vi "Update Monkeys Status.vi"(6 "Overwrite":bool, 7 "In ALL?":bool, 8 "error in (no error)":errorcluster, 9 "Status":T1, 10 "Monkey ID":string, 11 "Tamer in":refnum<class "Tamer.lvclass">=refnum) -> (0 "error out":errorcluster, 3 "Tamer out":refnum<class "Tamer.lvclass">)   [LabVIEW 2020, in "CIRCUS_uServices.lvlib" / "Tamer.lvlib" / "Tamer.lvclass"]
uses:
  Tamer.lvclass
  Monkey Summary.ctl
  Link Chain GUI.ctl
  TALOS/TALOS_PPL.lvlibp/Father of all uServices/Father of all uServices/Father of all uServices.lvclass
  TALOS/TALOS_PPL.lvlibp
  Run Utilities/TypeDefs/Monkey Status.ctl
  Run Utilities/Run Utilities.lvlib
  TALOS/TALOS_PPL.lvlibp/Father of all uServices/Father of all uServices/Children Methods/Get GUI Item Value - Variant.vi
  C:/Users/marco/Documents/GitHub_Lab/CIRCUS/TALOS/TALOS_PPL.lvlibp/Father of all uServices/Father of all uServices/Father of all uServices.lvclass
  C:/Users/marco/Documents/GitHub_Lab/CIRCUS/TALOS/TALOS_PPL.lvlibp/Ancestor/Ancestor/Ancestor.lvclass
  C:/Users/marco/Documents/GitHub_Lab/CIRCUS/TALOS/Actor Framework.lvlibp/1abvi3w/vi.lib/ActorFramework/Actor/Actor.lvclass
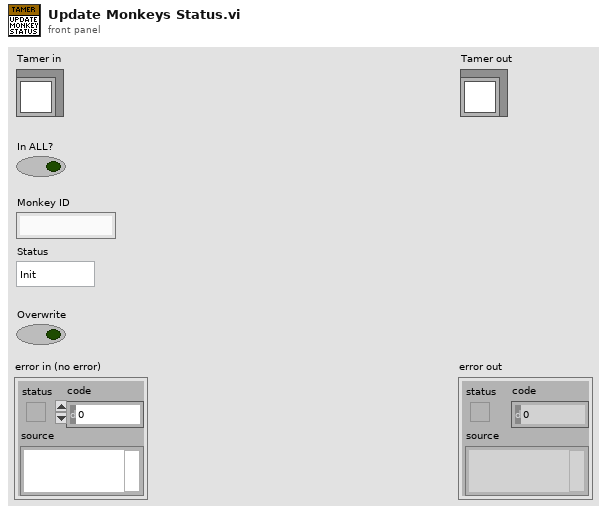
[diagram p1: front panel]
types:
  T1 = typedef "CIRCUS_uServices.lvlib/Run Utilities.lvlib/Monkey Status.ctl" = enum16{"Init", "Paused", "Ongoing", "Stopped", "Finished (no errors)", "Finished (with errors)"}
  T2 = typedef "CIRCUS_uServices.lvlib/Tamer.lvlib/Tamer.lvclass/Monkey Summary.ctl" = cluster{"Color":u32, "Status":T1, "Continuous":bool, "Scripts left":u32, "Scripts skipped":u32, "ETA":string, "Current Action":string, "Report from previous RUNs":string, "Monkey ID":string, "With DAQ?":bool, "Linked?":T3, "Paused":bool}
  T3 = typedef "CIRCUS_uServices.lvlib/Tamer.lvlib/Tamer.lvclass/Link Chain GUI.ctl" = bool
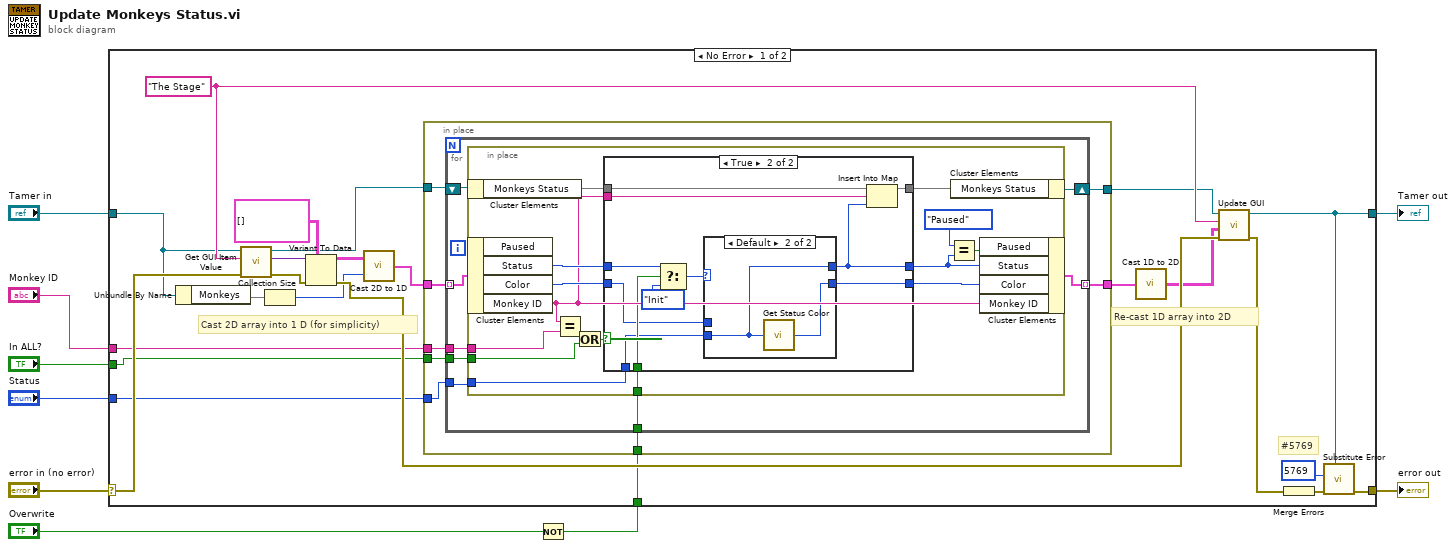
[diagram p0: block diagram]
diagram:
  n1 = Not(x="Overwrite") -> (.not. x?=w1:bool)
  n2 = case shown="No Error" "error in (no error)" {
    selector: "error in (no error)" -> [w28 w84]
    tunnel: [w33 w84] -> w8
    tunnel: [w32 w83] -> w6
    tunnel: "Tamer in" -> [w10 w83]
    tunnel: "Status" -> [w16 _]
    tunnel: "Monkey ID" -> [w15 _]
    tunnel: "In ALL?" -> [w14 _]
    tunnel: w1 -> [w11 _]
    frame No Error {
      w17 = "The Stage" ("FP Item Name")
      # "Re-cast 1D array into 2D"
      # "Cast 2D array into 1 D (for simplicity)"
      # "#5769"
      n3 = Unbundle By Name(w10) -> ("Monkeys"=w21:map{string, string[]})
      n4 = call-poly "Get GUI Item Value.vi"("error in (no error)"=w28, "FP Item Name"=w17, "uService Template in"=w10) -> ("error out"=w22:errorcluster, "Value"=w24:variant, "uService Template out"=w13:refnum<class "Tamer.lvclass">)  [unwired: 6 in]
      n5 = Collection Size(1:w21) -> (0:w20:i32)
      n6 = Variant To Data(error in=w22, type=T2[][] [] ("2D Synchronous Monkeys"), Variant=w24) -> (data=w23:T2[][], error out=w26:errorcluster)
      n7 = call "Cast 2D to 1D.vi"("1D size"=w20, "2D Synchronous Monkeys"=w23) -> ("1D Synchronous Monkeys"=w27:T2[])
      n8 = in-place {
        in-place-border: w27 -> [w41]
        in-place-border: [w40] -> w25
        in-place-border: w16 -> [w37]
        in-place-border: w15 -> [w39]
        in-place-border: w14 -> [w38]
        in-place-border: w13 -> [w36]
        in-place-border: [w35] -> w12
        in-place-border: w11 -> [w34]
        n9 = for {
          tunnel: w41 -> [w49] mode=indexing
          tunnel: w37 -> [w48]
          tunnel: [w47] -> w40 mode=indexing
          tunnel: w39 -> [w46]
          tunnel: w38 -> [w45]
          shift-right: [w43] -> w35
          shift-left: w36 -> [w44]
          tunnel: w34 -> [w42]
          n10 = in-place {
            in-place-border: w48 -> [w64]
            in-place-border: w46 -> [w63]
            in-place-border: w45 -> [w60]
            in-place-border: w42 -> [w53]
            n11 = in-place-cluster #1(w44) -> ("Monkeys Status"=w56:map{string, T1})
            n12 = in-place-cluster #2(w49) -> ("Status"=w59:T1, "Color"=w57:u32, "Monkey ID"=w54:string)  [unwired: 1 out]
            n13 = Equal?(x=w54, y=w63) -> (x = y?=w61:bool)
            n14 = Or(x=w61, y=w60) -> (x .or. y?=w62:bool)
            n15 = case shown="True" w62 {
              tunnel: [w66 w70] -> w58
              tunnel: w64 -> [_ w71]
              tunnel: w59 -> [w67 w75]
              tunnel: [w67 w69] -> w52
              tunnel: w57 -> [w66 w68]
              tunnel: w56 -> [w65 w78]
              tunnel: [w65 w77] -> w55
              tunnel: w54 -> [_ w76]
              tunnel: w53 -> [_ w74]
              frame False {
              }
              frame True {
                n16 = Select(t=w75, s=w74, f=Monkey_Status."Init") -> (s? t:f=w72:T1)
                n17 = case shown="Default" w72 {
                  selector: w72 -> [w79 _]
                  tunnel: w71 -> [_ w81]
                  tunnel: [w80 w82] -> w70
                  tunnel: [w79 w81] -> w69
                  tunnel: w68 -> [w80 _]
                  frame "Stopped".."Finished (with errors)" {
                  }
                  frame Default {
                    n18 = call "Get Status Color.vi"("Monkey Status"=w81) -> ("Color"=w82:u32)
                  }
                }
                n19 = Insert Into Map(map in=w78, key=w76, value=w69) -> (map out=w77:map{string, T1})  [unwired: 2 out]
              }
            }
            n20 = Equal?(x=Monkey_Status."Paused", y=w52) -> (x = y?=w50:bool)
            n21 = in-place-cluster #1("Monkeys Status"=w55) -> (w43:refnum<class "Tamer.lvclass">)
            n22 = in-place-cluster #2("Paused"=w50, "Status"=w52, "Color"=w58, "Monkey ID"=w54) -> (w47:T2)
          }
        }
      }
      n23 = call "Cast 1D to 2D.vi"("1D Monkeys"=w25) -> ("2D Monkeys"=w18:T2[][])
      n24 = call "Update GUI.vi"("error in (no error)"=w26, "Data"=w18, "GUI Item Name"=w17, "uService Template in"=w12) -> ("error out"=w30:errorcluster, "uService Template out"=w32:refnum<class "Tamer.lvclass">)  [unwired: 6 in]
      n25 = Merge Errors(w30) -> (w29:errorcluster)
      n26 = call "Substitute Error.vi"("LabVIEW Object"=w32, "error in (no error)"=w29, "Error Code"=5769) -> ("error out"=w33:errorcluster)  [unwired: 8 in]
    }
    frame Error {
    }
  }
  "error out" <- w8
  "Tamer out" <- w6
